vi "SSC DCPower Query Output State.vi"(0 "DCPower SSC in":T2[](array[typedef]), 5 "Output State":T1 items=["Constant Voltage", "Constant Current"], 11 "error in":errorcluster) -> (4 "DCPower SSC out":T2[](array[typedef]), 6 "In State?":bool[](array[boolean]), 15 "error out":errorcluster)   [LabVIEW 2019]
doc: "Queries the specified output channel to determine if the output channels are currently in the state specified by <B>output state</B>."
uses:
  SSC DCPower.ctl
  <instrlib>/niDCPower/nidcpower.llb/niDCPower Output State.ctl
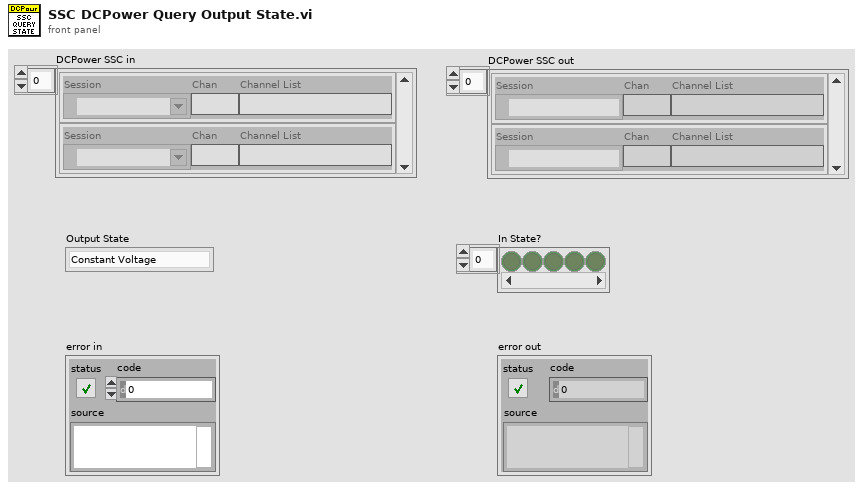
[diagram p1: front panel]
types:
  T1 = typedef "niDCPower Output State.ctl" = u16
  T2 = typedef "SSC DCPower.ctl" = cluster{"Session":refnum<k15>, "Chan":string, "Channel List":string}
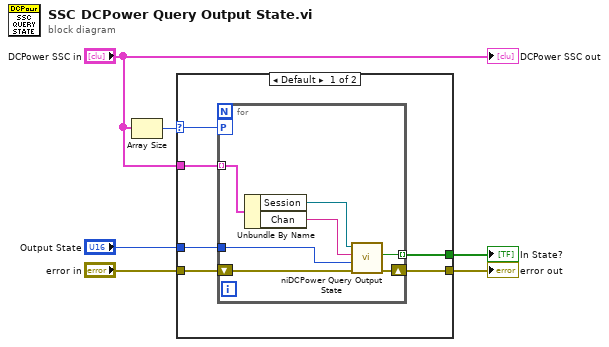
[diagram p0: block diagram]
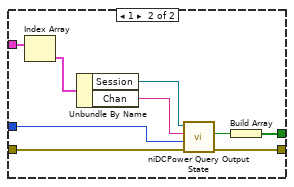
[diagram p2: hidden frame]
diagram:
  n1 = Array Size(array="DCPower SSC in") -> (size(s)=w2:i32)
  n2 = case shown="Default" w2 {
    selector: w2 -> [w8 _]
    tunnel: [w12 w28] -> w6
    tunnel: [w11 w20] -> w5
    tunnel: "error in" -> [w10 w26]
    tunnel: "Output State" -> [w9 w25]
    tunnel: "DCPower SSC in" -> [w7 w24]
    frame Default {
      n3 = for {
        tunnel: w7 -> [w19] mode=indexing
        tunnel: [w16] -> w11 mode=indexing
        workers-P: w8 -> [_]
        tunnel: w9 -> [w15]
        shift-right: [w17] -> w12
        shift-left: w10 -> [w18]
        n4 = Unbundle By Name(w19) -> ("Session"=w14:refnum<k15>, "Chan"=w13:string)
        n5 = call <instrlib>:"niDCPower Query Output State.vi"("error in (no error)"=w18, "output state"=w15, "channel name"=w13, "instrument handle"=w14) -> ("error out"=w17:errorcluster, "in state?"=w16:bool)  [unwired: 5 in, 1 out]
      }
    }
    frame 1 {
      n6 = Index Array(array=w24) -> (element=w21:T2)  [unwired: 1 in]
      n7 = Unbundle By Name(w21) -> ("Session"=w23:refnum<k15>, "Chan"=w22:string)
      n8 = call <instrlib>:"niDCPower Query Output State.vi"("error in (no error)"=w26, "output state"=w25, "channel name"=w22, "instrument handle"=w23) -> ("error out"=w28:errorcluster, "in state?"=w27:bool)  [unwired: 5 in, 1 out]
      n9 = Build Array(w27) -> (w20:bool[])
    }
  }
  "error out" <- w6
  "In State?" <- w5
  "DCPower SSC out" <- "DCPower SSC in"
